vi "ActDriveStraight.vi"(9 "FirstTime":bool, 10 "MaxSpeed (ft/s)":dbl, 11 "Dist (ft)":dbl) -> (1 "XSpeedDemand":dbl, 3 "Done":bool)   [LabVIEW 2023]
doc: "Robot will drive forward straight a set distance utilizing position control \n\nInputs:\n-- MaxSpeed -- Double -- in ft/s, the MaxSpeed the robot can go -- \n-- Dist (ft) -- Double -- Distance in feet you want the robot to go -- \n-- FirstTime -- Boolean -- Input true the first time this function is called, sets the target position -- \n\nOutputs:\n-- Done -- Bool -- has the robot reached its target distance\n-- LeftSpeedDemand -- Double -- Speed Demand for left drive train inorder to reach target -- \n-- RightSpeedDemand -- Double -- Speed Demand for left drive train inorder to reach target --"
uses:
  <vilib>/Rock Robotics/Network Tables/NT Write Number.vi
  <vilib>/Rock Robotics/WPI/ThirdParty/JAS_Junk/TrajLib/Trajectory_Library.lvlib
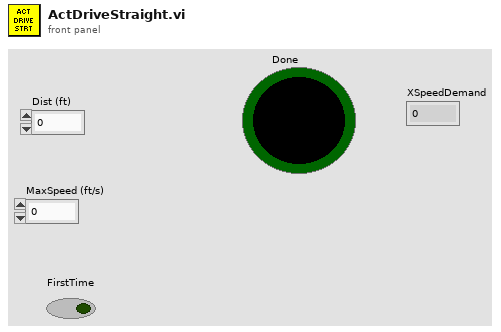
[diagram p1: front panel]
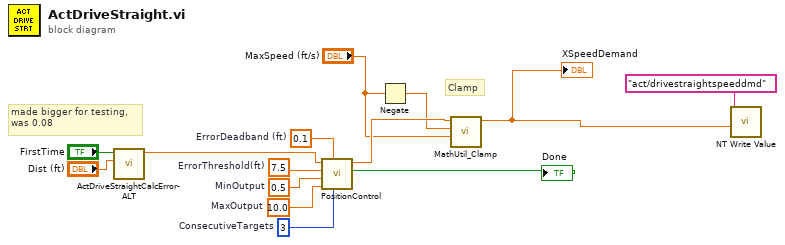
[diagram p0: block diagram]
diagram:
  w5 = 10.0  # MaxOutput
  w6 = 0.5  # MinOutput
  w10 = 3  # ConsecutiveTargets
  w11 = 0.1  # ErrorDeadband (ft)
  w12 = 7.5  # ErrorThreshold(ft)
  # "made bigger for testing, \nwas 0.08"
  # "Clamp"
  n1 = call "ActDriveStraightCalcError-ALT.vi"("Dist (ft)"="Dist (ft)", "FirstTime"="FirstTime") -> ("Dist Error (Ft)"=w3:dbl)  [unwired: 9 in]
  n2 = call "PositionControl.vi"("ConsecutiveTargets"=w10, "ErrorDeadband"=w11, "MaxOutput"=w5, "MinOutput"=w6, "ErrorThreshold"=w12, "Error"=w3) -> ("OnTarget"=→"Done":bool, "OutputValue"=w9:dbl)  [unwired: 3 in, 1 out]
  n3 = Negate(x="MaxSpeed (ft/s)") -> (-x=w8:dbl)
  n4 = call <vilib>:"MathUtil_Clamp.vi"("High Limit"="MaxSpeed (ft/s)", "Low Limit"=w8, "Value"=w9) -> ("Result"=w2:dbl)  [unwired: 8 in]
  "XSpeedDemand" <- w2
  n5 = call-poly <vilib>:"NT Write Value.vi"("value"=w2, "name"="act/drivestraightspeeddmd") -> ()  [unwired: 9 in, 1 out]
